vi "WriteRead Data.vi"(6 "NoStop (F)":bool, 7 "I2C Device in":refnum<class "I2C Peripheral.lvclass">, 8 "error in (no error)":errorcluster, 9 "Len":u8, 10 "Write Data":string, 11 "Session In":refnum<class "Session.lvclass">) -> (0 "error out":errorcluster, 1 "Read Data":string, 3 "Session Out":refnum<class "Session.lvclass">)   [LabVIEW 2020, in "CTI.lvlib" / "I2C Peripheral.lvclass"]
uses:
  I2C Peripheral.lvclass
  I2C Peripheral.lvclass/I2C Peripheral.ctl
  I2C/I2C.lvclass
  Session/Session.lvclass
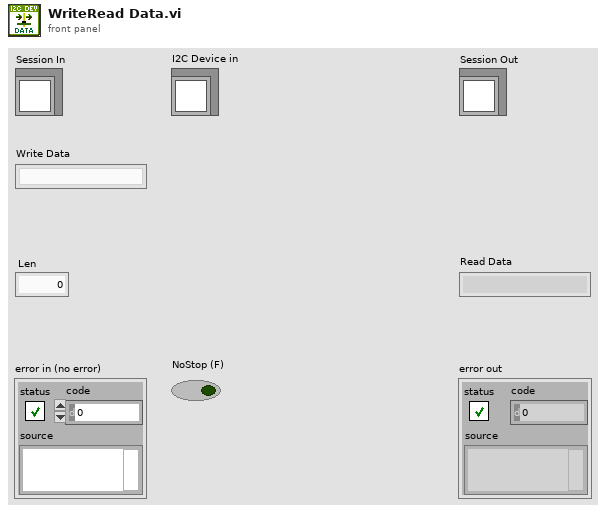
[diagram p1: front panel]
types:
  T1 = typedef "CTI.lvlib/I2C Address.ctl" = u8
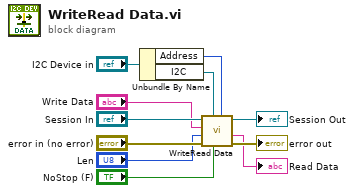
[diagram p0: block diagram]
diagram:
  n1 = Unbundle By Name("I2C Device in") -> ("Address"=w5:T1, "I2C"=w6:refnum<class "I2C.lvclass">)
  n2 = call "WriteRead Data.vi"("Address"=w5, "NoStop (F)"="NoStop (F)", "I2C"=w6, "error in (no error)"="error in (no error)", "Len"="Len", "Write Data"="Write Data", "Session In"="Session In") -> ("error out"=→"error out":errorcluster, "Read Data"=→"Read Data":string, "Session Out"=→"Session Out":refnum<class "Session.lvclass">)  [unwired: 2 in]
